vi "Volt_Out_사인파에 의한.vi"() -> ()   [LabVIEW 2018]
uses:
  <vilib>/DAQmx/miscellaneous.llb/DAQmx Fill In Error Info.vi
  <vilib>/DAQmx/write.llb/DAQmx Write (Analog Wfm 1Chan NSamp).vi
  <vilib>/DAQmx/create/channels.llb/DAQmx Create Channel (AO-Voltage-Basic).vi
  <vilib>/DAQmx/configure/timing.llb/DAQmx Timing (Sample Clock).vi
  <vilib>/measure/NI_MABase.lvlib
  <resource>/objmgr/daqmx.rc
panel:
  out "웨이브폼 차트":waveform(dbl)(graph)
  in  "frequency":dbl=10.0 caption="주파수" format="%0.2p"
  in  "정지":bool
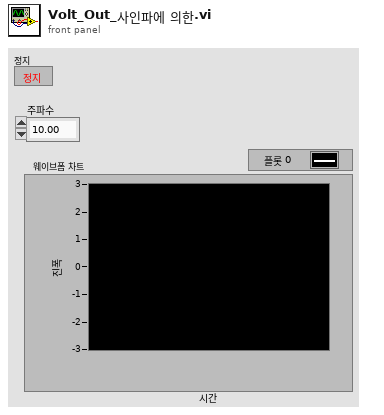
[diagram p1: front panel]
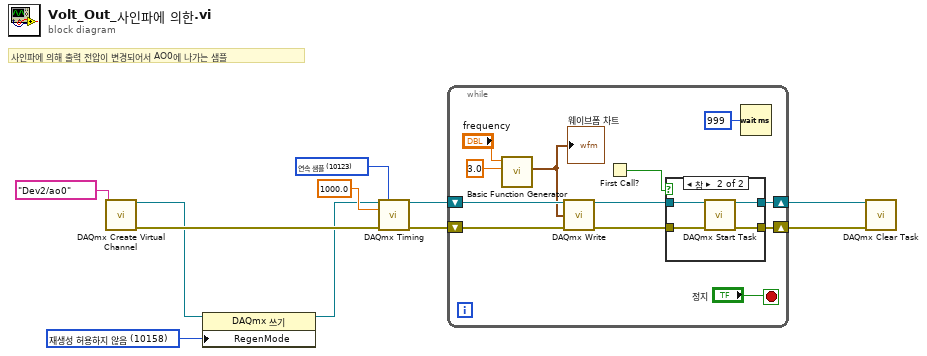
[diagram p0: block diagram]
diagram:
  w3 = 10158 items=["재생성 허용"=10097, "재생성 허용하지 않음"=10158] ("재생성 모드")
  w5 = 10123 items=["유한 샘플"=10178, "연속 샘플"=10123, "하드웨어 타이밍에 의한 단일 포인트"=12522] ("sample mode")
  # "사인파에 의해 출력 전압이 변경되어서 AO0에 나가는 샘플"
  n1 = call-poly <vilib>:"DAQmx Create Virtual Channel.vi"("physical channels"=tag "Dev2/ao0") -> ("task out"=w2:refnum<k21>, "error out"=w11:errorcluster)  [unwired: 13 in]
  n2 = property class="DAQmx 쓰기"(reference=w2, "RegenMode"=w3) -> (reference out=w1:refnum<k21>)  [unwired: 1 in, 1 out]
  n3 = call-poly <vilib>:"DAQmx Timing.vi"("task/channels in"=w1, "sample mode"=w5, "rate"=1000.0, "error in"=w11) -> ("task out"=w10:refnum<k21>, "error out"=w9:errorcluster)  [unwired: 10 in]
  n4 = while {
    shift-right: [w19] -> w8
    shift-left: w10 -> [w23]
    shift-right: [w18] -> w7
    shift-left: w9 -> [w22]
    stop <- "정지" stop-if-true
    n5 = call <vilib>:"Basic Function Generator.vi"("amplitude"=3.0, "frequency"="frequency") -> ("signal out"=w13:waveform(dbl))  [unwired: 7 in, 2 out]
    "웨이브폼 차트" <- w13
    n6 = call-poly <vilib>:"DAQmx Write.vi"("task/channels in"=w23, "data"=w13, "error in"=w22) -> ("task out"=w21:refnum<k21>, "error out"=w20:errorcluster)  [unwired: 10 in, 1 out]
    n7 = First Call?() -> (First Call?: T/F=w16:bool)
    n8 = case shown="참" w16 {
      tunnel: w21 -> [w25 w29]
      tunnel: w20 -> [w24 w28]
      tunnel: [w25 w27] -> w19
      tunnel: [w24 w26] -> w18
      frame False {
      }
      frame True {
        n9 = call <vilib>:"DAQmx Start Task.vi"("task/channels in"=w29, "error in"=w28) -> ("task out"=w27:refnum<k21>, "error out"=w26:errorcluster)  [unwired: 12 in]
      }
    }
    n10 = Wait (ms)(milliseconds to wait=u32 999 ("대기 시간 (ms)")) -> ()  [unwired: 1 out]
  }
  n11 = call <vilib>:"DAQmx Clear Task.vi"("task in"=w8, "error in"=w7) -> ()  [unwired: 13 in, 1 out]
